vi "DriveSync.vi"   [LabVIEW 2012]
uses:
  Controls/StateCtrl.ctl
types:
  T1 = typedef "StateCtrl.ctl" = enum16{"Init", "Idle", "Stop"}
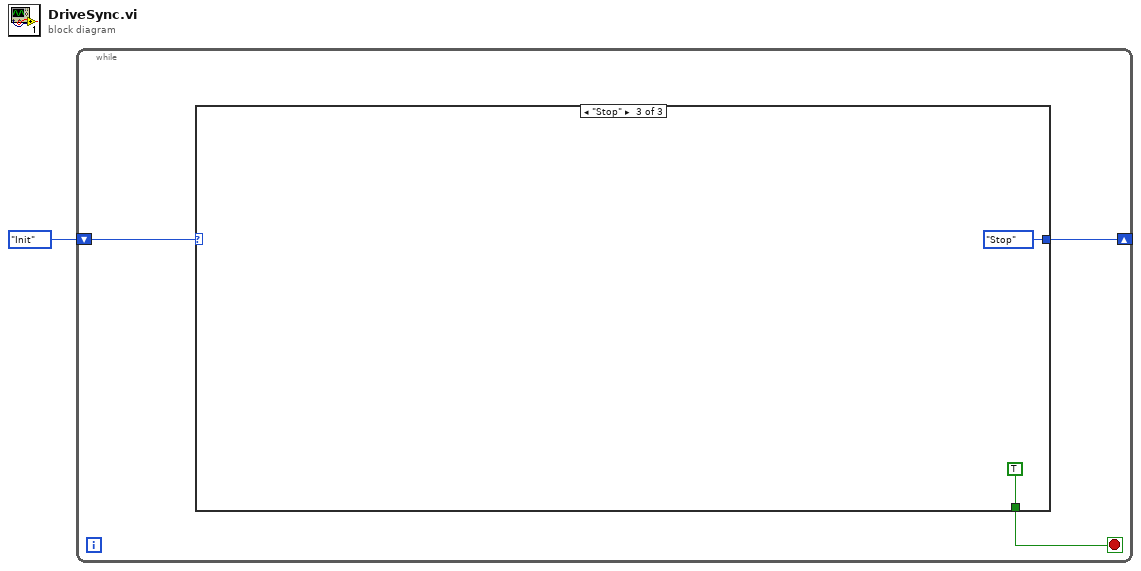
[diagram p0: block diagram]
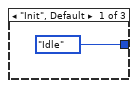
[diagram p2: hidden frame]
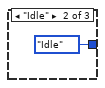
[diagram p3: hidden frame]
diagram:
  n1 = while {
    shift-right: [w3] -> _
    shift-left: StateCtrl."Init" -> [w4]
    stop <- w2 stop-if-true
    n2 = case shown="\"Stop\"" w4 {
      tunnel: [StateCtrl."Idle" StateCtrl."Idle" StateCtrl."Stop"] -> w3
      tunnel: [_ _ TRUE] -> w2
      frame "Init", Default {
      }
      frame "Idle" {
      }
      frame "Stop" {
      }
    }
  }
